vi "mks670_set_pressure.vi"() -> ()   [LabVIEW 2019]
panel:
  out "Command Read":string
  out "tpg361_visa 3":refnum<visa-resource-name>
  out "err_out 2":errorcluster
  out "Status":bool
  in  "tpg361_b2r":u32
  in  "err_in":errorcluster
  in  "tpg361_delay":u32=500
  in  "tpg361_visa":refnum<visa-resource-name>
  # "VISA"
  # "DELAY"
  # "BYTE AT PORT"
  # "STATUS"
  # "ERROR"
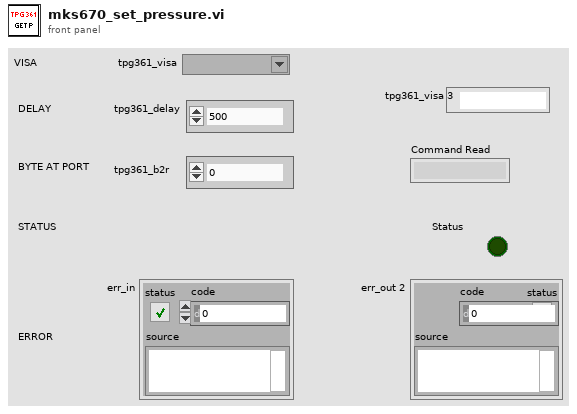
[diagram p1: front panel]
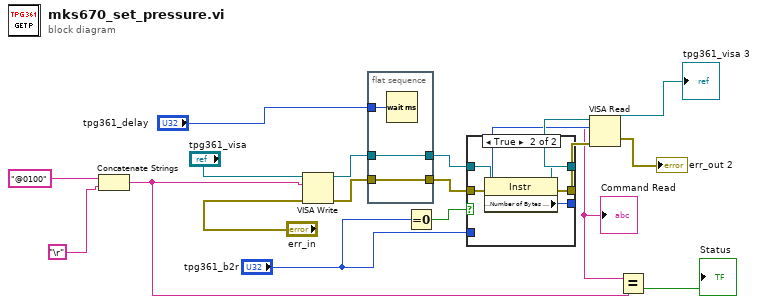
[diagram p0: block diagram]
diagram:
  n1 = Concatenate Strings("@0100" ("string"), "\r") -> (w1:string)
  n2 = VISA Write(VISA resource name="tpg361_visa", write buffer=w1, error in (no error)="err_in") -> (VISA resource name out=w17:refnum<visa-resource-name>, error out=w19:errorcluster)  [unwired: 1 out]
  n3 = flat-sequence {
    tunnel: w19 -> [w21]
    tunnel: [w21] -> w18
    tunnel: w17 -> [w20]
    tunnel: [w20] -> w16
    tunnel: "tpg361_delay" -> [w22]
    frame #0 {
      n4 = Wait (ms)(milliseconds to wait=w22) -> ()  [unwired: 1 out]
    }
  }
  n5 = Equal To 0?(x="tpg361_b2r") -> (x = 0?=w12:bool)
  n6 = case shown="True" w12 {
    tunnel: w18 -> [w24 w30]
    tunnel: w16 -> [w25 w29]
    tunnel: [w25 w28] -> w10
    tunnel: [w24 w27] -> w9
    tunnel: [w23 w26] -> w8
    tunnel: "tpg361_b2r" -> [w23 _]
    frame False {
    }
    frame True {
      n7 = property class="Instr"(reference=w29, error in=w30) -> (reference out=w28:refnum<visa-resource-name>, error out=w27:errorcluster, "Serial Settings:Number of Bytes at Serial Port"=w26:u32)
    }
  }
  n8 = VISA Read(VISA resource name=w10, byte count=w8, error in (no error)=w9) -> (VISA resource name out=→"tpg361_visa 3":refnum<visa-resource-name>, read buffer=w6:string, error out=→"err_out 2":errorcluster)  [unwired: 1 out]
  "Command Read" <- w6
  n9 = Equal?(x=w6, y=w1) -> (x = y?=→"Status":bool)
